vi "write station hall config noSCU.vi"(4 "name":string[](array[string]), 6 "section":string="Hall Counts", 8 "error in":errorcluster, 10 "value":i32[](array[numeric]), 11 "configuration file path in":path) -> (0 "error out":errorcluster, 3 "configuration file path out":path)   [LabVIEW 2018]
uses:
  05.UserVI's/file io/ini/type defs/ini file actions.ctl
  05.UserVI's/file io/ini/type defs/ini entry types.ctl
  05.UserVI's/file io/ini/type defs/ini entry value.ctl
  05.UserVI's/file io/ini/type defs/ini entry.ctl
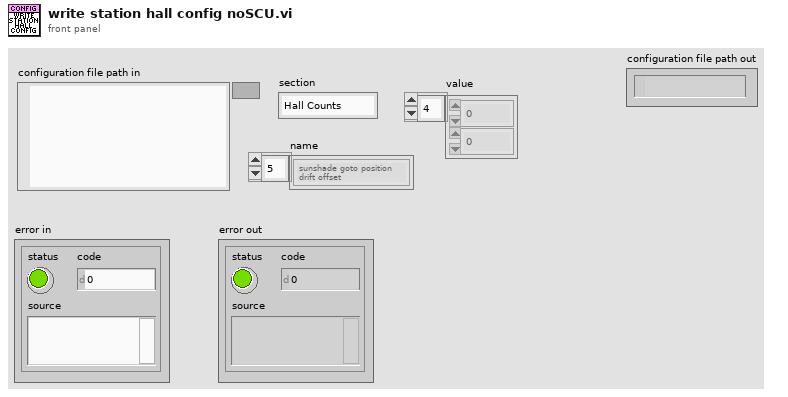
[diagram p1: front panel]
types:
  T1 = typedef "ini entry value.ctl" = cluster{"Boolean":bool, "Dbl":dbl, "I32":i32, "Path":path, "String":string, "U32":u32}
  T2 = typedef "ini entry types.ctl" = enum16{"Boolean", "Double", "I32", "Path", "String", "U32"}
  T3 = typedef "ini file actions.ctl" = enum16{"read ini", "write ini"}
  T4 = typedef "ini entry.ctl" = cluster{"section":string, "key":string, "type":T2, "default value":T1}
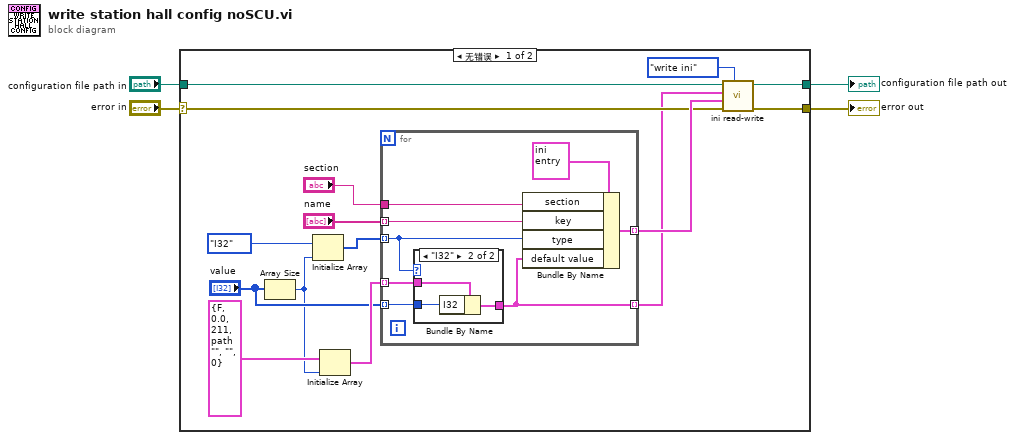
[diagram p0: block diagram]
diagram:
  n1 = case shown="无错误" "error in" {
    selector: "error in" -> [w14 w33]
    tunnel: "configuration file path in" -> [w19 w32]
    tunnel: [w17 w32] -> w3
    tunnel: [w13 w33] -> w2
    frame No Error {
      n2 = Array Size(array="value") -> (size(s)=w6:i32)
      n3 = Initialize Array(ini_entry_types."I32" ("type"), w6) -> (w10:T2[])
      n4 = Initialize Array(T1 {"Boolean"=FALSE, "Dbl"=0.0, "I32"=211, "Path"=path "", "String"="", "U32"=0} ("default value"), w6) -> (w8:T1[])
      n5 = for {
        tunnel: "section" -> [w26]
        tunnel: "name" -> [w25] mode=indexing
        tunnel: w10 -> [w23] mode=indexing
        tunnel: w8 -> [w22] mode=indexing
        tunnel: [w24] -> w15 mode=indexing
        tunnel: "value" -> [w21] mode=indexing
        tunnel: [w20] -> w5 mode=indexing
        n6 = case shown="\"I32\"" w23 {
          tunnel: w22 -> [w28 w31]
          tunnel: w21 -> [_ w30]
          tunnel: [w28 w29] -> w20
          frame "Boolean", Default {
          }
          frame "I32" {
            n7 = Bundle By Name(cluster=w31, "I32"=w30) -> (w29:T1)
          }
        }
        n8 = Bundle By Name(cluster=T4 {"section"="", "key"="", "type"=enum."Boolean", "default value"={"Boolean"=FALSE, "Dbl"=0.0, "I32"=0, "Path"=path "", "String"="", "U32"=0}}, "section"=w26, "key"=w25, "type"=w23, "default value"=w20) -> (w24:T4)
      }
      n9 = call "ini read-write.vi"("action"=ini_file_actions."write ini", "error in (no error)"=w14, "ini entry descriptors"=w15, "values in"=w5, "configuration file path"=w19) -> ("error out"=w13:errorcluster, "configuration file path out"=w17:path)  [unwired: 4 in, 1 out]
    }
    frame Error {
    }
  }
  "configuration file path out" <- w3
  "error out" <- w2
